vi "File Handling - Create filenames.vi"(8 "error in":errorcluster) -> (0 "error out":errorcluster, 1 "Active Run":bool, 2 "Binary Logfile path":path, 3 "ASCII Logfile path":path)   [LabVIEW 2011]
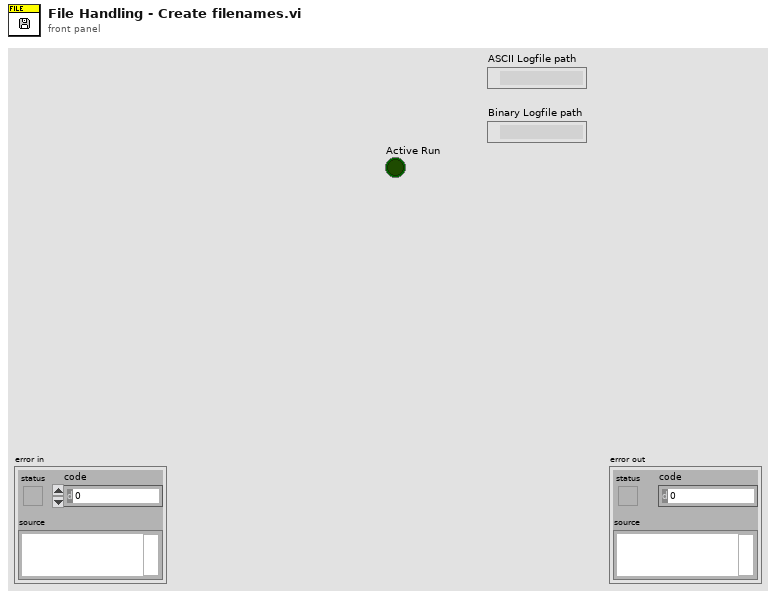
[diagram p1: front panel]
types:
  T1 = typedef "Project infor with project path.ctl" = cluster{"Project path":path, "data":T2, "Comment":string}
  T2 = typedef "Project in icluster.ctl" = cluster{"Job and Site":T3, "Tool":T5, "Run Information":T6}
  T3 = typedef "Job and site cluster.ctl" = cluster{"Project Number":string, "Client Company":string, "Country":T4, "Field":string, "Rig":string, "Well":string}
  T4 = typedef "List of all contrys(combo box).ctl" = string
  T5 = typedef "Tool registration ID.ctl" = cluster{"Tractor type":string, "Tool":string, "Serial #":string}
  T6 = typedef "Run Information.ctl" = cluster{"Active Run":bool, "String Check Rec":bool, "Run Number":i32, "Time of File Start":string}
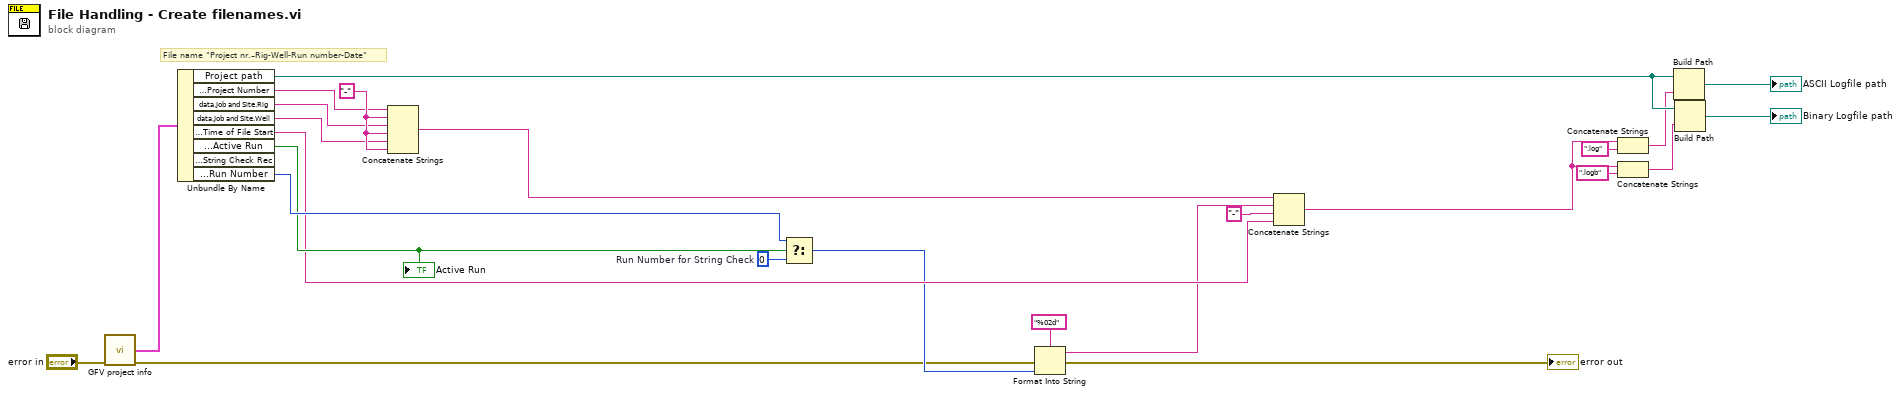
[diagram p0: block diagram]
diagram:
  w8 = 0  # Run Number for String Check
  w21 = "-"
  # "File name \"Project nr.–Rig-Well-Run number-Date\""
  n1 = call "GFV project info.vi"("error in (no error)"="error in") -> ("Project info out"=w11:T1, "error out"=w2:errorcluster)  [unwired: 13 in]
  n2 = Unbundle By Name(w11) -> ("Project path"=w25:path, "data.Job and Site.Project Number"=w18:string, "data.Job and Site.Rig"=w19:string, "data.Job and Site.Well"=w20:string, "data.Run Information.Time of File Start"=w6:string, "data.Run Information.Active Run"=w7:bool, "data.Run Information.Run Number"=w9:i32)  [unwired: 1 out]
  "Active Run" <- w7
  n3 = Concatenate Strings(w18, w21, w19, w21, w20, w21) -> (w15:string)
  n4 = Select(t=w9, s=w7, f=w8) -> (s? t:f=w4:i32)
  n5 = Format Into String(format string="%02d", error in=w2, w4) -> (resulting string=w3:string, error out=→"error out":errorcluster)  [unwired: 1 in]
  n6 = Concatenate Strings(w15, w3, "-", w6) -> (w14:string)
  n7 = Concatenate Strings(w14, ".log" ("string")) -> (w23:string)
  n8 = Concatenate Strings(w14, ".logb" ("string")) -> (w24:string)
  n9 = Build Path(base path=w25, name or relative path=w23) -> (appended path=→"ASCII Logfile path":path)
  n10 = Build Path(base path=w25, name or relative path=w24) -> (appended path=→"Binary Logfile path":path)
